vi "CheckFPGABitfileRequirements.vi"(8 "error in (no error)":errorcluster) -> (0 "error out":errorcluster, 1 "system info":T1, 2 "description":string, 3 "bitfile dir":path, 5 "valid":bool)   [LabVIEW 2017, in "FpgaBitfileManager.lvlib"]
uses:
  <vilib>/addons/InsightCM/Devices/Shared/Common/FpgaBitfileManager/FpgaBitfileManager.lvlib
  <vilib>/addons/cRIODetectHW/control/SystemHW.ctl
  <vilib>/addons/cRIODetectHW/control/cRIO Product Info.ctl
  <vilib>/addons/InsightCM/Utilities/GlobalConfiguration/GlobalConfiguration.lvlib
  <vilib>/addons/SystemInfoProcess/SystemInfoProcess.lvlib
  <vilib>/addons/InsightCM/Devices/Shared/Cms/CmsFpgaBitfileManager/CmsFpgaBitfileManager.lvlib
  <vilib>/addons/cRIODetectHW/cRIODetectHW.lvlib
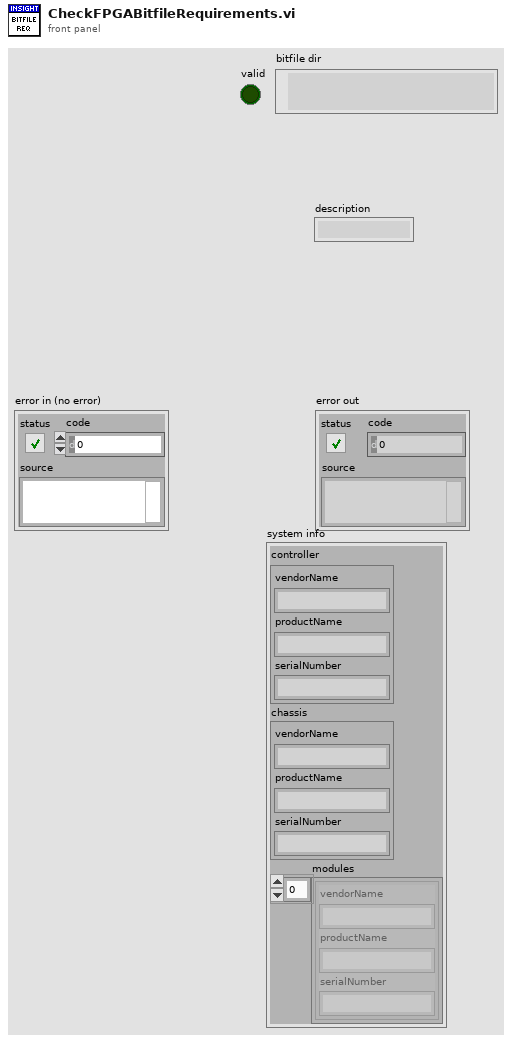
[diagram p1: front panel]
types:
  T1 = typedef "cRIODetectHW.lvlib/SystemHW.ctl" = cluster{"controller":T2, "chassis":T2, "modules":T2[]}
  T2 = typedef "cRIODetectHW.lvlib/cRIO Product Info.ctl" = cluster{"vendorName":string, "productName":string, "serialNumber":string}
  T3 = typedef "R2_Device.ctl" = cluster{"Id":string, "Name":string, "DeviceType":string, "HardwareName":string, "IpAddress":string, "HardwareInfo":T4[], "ApplicationType":string, "ApplicationVersion":string, "EquipmentIds":string[], "ConfigurationVersion":string, "State":T5, "Properties":T4[], "DataGroups":T6[], "BurstModeTrigger":T10}
  T4 = typedef "KeyValuePair.ctl" = cluster{"Key":string, "Value":string}
  T5 = typedef "DeviceState.ctl" = cluster{"Disabled":bool}
  T6 = typedef "R2_DataGroup.ctl" = cluster{"Name":string, "OperatingStates":T7[], "Properties":T4[], "EquipmentIds":string[], "AssetNodeId":string}
  T7 = typedef "OperatingState.ctl" = cluster{"Name":string, "Properties":T4[], "Triggers":T8[]}
  T8 = typedef "Trigger.ctl" = cluster{"Type":string, "Expression":string, "Conditions":T9[]}
  T9 = typedef "Condition.ctl" = cluster{"Source":string, "Type":string, "Operator":string, "CompareTo":string, "DwellSeconds":dbl}
  T10 = typedef "BurstModeTrigger.ctl" = cluster{"Trigger":T8, "SampleRate":string, "AcquisitionLength":string}
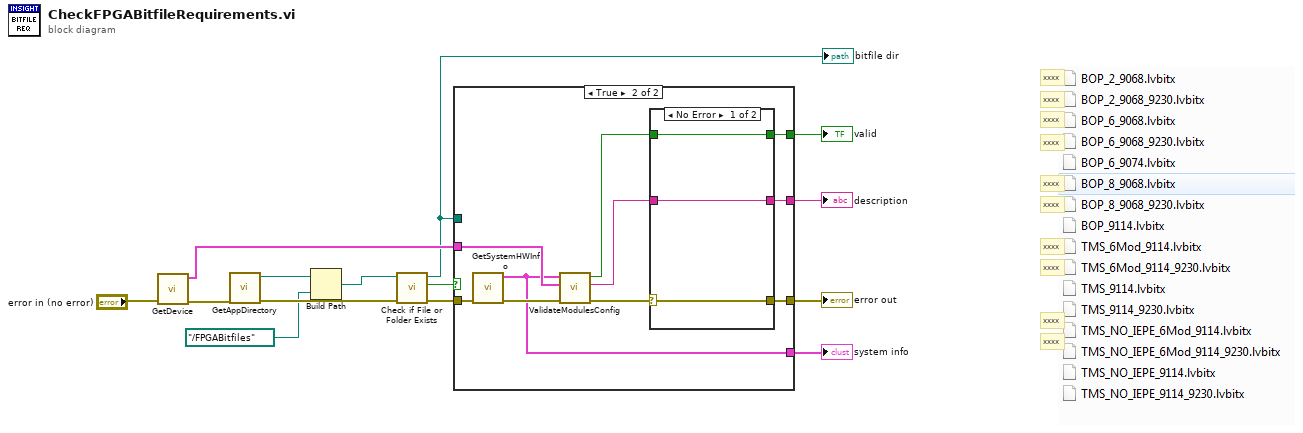
[diagram p0: block diagram]
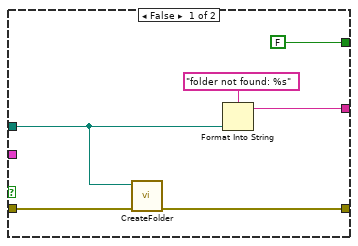
[diagram p2: hidden frame]
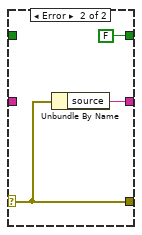
[diagram p3: hidden frame]
diagram:
  # "xxxx"
  # "xxxx"
  # "xxxx"
  # "xxxx"
  # "xxxx"
  # "xxxx"
  # "xxxx"
  # "xxxx"
  # "xxxx"
  # "xxxx"
  n1 = call <vilib>:"GetDevice.vi"("error in (no error)"="error in (no error)") -> ("error out"=w7:errorcluster, "device configuration"=w6:T3)  [unwired: 8 in, 1 out]
  n2 = call <vilib>:"GetAppDirectory.vi"("error in (no error)"=w7) -> ("error out"=w14:errorcluster, "application directory"=w13:path)  [unwired: 9 in]
  n3 = Build Path(base path=w13, name or relative path=path "../FPGABitfiles" ("application directory")) -> (appended path=w12:path)
  n4 = call <vilib>:"Check if File or Folder Exists.vi"("error in (no error)"=w14, "path"=w12) -> ("error out"=w10:errorcluster, "file or folder exists?"=w11:bool, "dup path"=w2:path)  [unwired: 7 in]
  "bitfile dir" <- w2
  n5 = case shown="True" w11 {
    tunnel: w10 -> [w16 w30]
    tunnel: w2 -> [w17 _]
    tunnel: [w15 w27] -> w9
    tunnel: w6 -> [_ w28]
    tunnel: [FALSE ("valid") w26] -> w5
    tunnel: [w18 w23] -> w3
    tunnel: [_ w21] -> w1
    frame False {
      n6 = call <vilib>:"CreateFolder.vi"("error in (no error)"=w16, "folder"=w17) -> ("error out"=w15:errorcluster)  [unwired: 8 in, 1 out]
      n7 = Format Into String(format string="folder not found: %s", w17) -> (resulting string=w18:string)  [unwired: 2 in, 1 out]
    }
    frame True {
      n8 = call <vilib>:"GetSystemHWInfo.vi"("error in (no error)"=w30) -> ("error out"=w29:errorcluster, "system info"=w21:T1)  [unwired: 8 in, 1 out]
      n9 = call <vilib>:"ValidateModulesConfig.vi"("error in (no error)"=w29, "Device"=w28, "system info"=w21) -> ("error out"=w22:errorcluster, "description"=w24:string, "valid"=w25:bool)  [unwired: 6 in]
      n10 = case shown="No Error" w22 {
        selector: w22 -> [w33 w36]
        tunnel: [w33 w36] -> w27
        tunnel: [w32 FALSE ("valid")] -> w26
        tunnel: w25 -> [w32 _]
        tunnel: [w31 w35] -> w23
        tunnel: w24 -> [w31 _]
        frame No Error {
        }
        frame Error {
          n11 = Unbundle By Name(w36) -> ("source"=w35:string)
        }
      }
    }
  }
  "error out" <- w9
  "valid" <- w5
  "description" <- w3
  "system info" <- w1
